vi "FGV Spans abarbeiten.vi"(5 "running":bool, 6 "Aktion":T10, 8 "error in (no error)":errorcluster caption="Fehler (Eingang, kein Fehler)", 11 "SpanInletClusterArray in":T1[](array[typedef]) {"zusätzliche Zeitdauer Erster Punkt" min=30 step=1 format="%#_5g"; "Zeitdauer Stufen" format="%#_5g"; "Max Fehler" format="%#_5g"; "Anzahl Stufen" format="%#_5g"; "Komponenten"."Komponente 5"."Komponente:" items=["NO (350,3000) LP 191C", "NO2 (150) LP 191C (1of2)", "NO2 (2000) LP 191C (2of2)", "N2O (300) LP 191C (1of2)", "NH3 (300) LP 191C (1of2)", "NH3 (900,3000) LP 191C (2of2)", "HNCO (400) 191C", "H2O% (30) LP 191C", "Formaldehyde (70,500) LP 191C", "CO2 low% (4) LP 191C (2of2)", "CO2% (20) LP 191C (1of2)", "CO (700) LP 191C (1of3)", "CO% (1) LP 191C (2of3)", "Propylene (1000) LP 191C", "Aromatic HC C7 (500) LP 191C", "Ethylene (1000) LP 191C", "CH4 (250) LP 191C (1of2)", "CH4 (5000) LP 191C (2of2)", "Ethane (1000) LP 191C", "Acetylene (1000) LP 191C", "HNO2 (20) 191C", "MeOH (1000) 191C", "CO% (10) LP 191C (3of3)", "Formic Acid (100) 191C", "SO2 (500) LP 191C", "Acetaldehyde (1000) LP 191C", "COS (100) LP 191C", "1,3 butadiene (100) LP 191C", "Oil as Octane (200) LP 191C", "N2O (1000) LP 191C (2of2)", "Propane (200) LP 191C", "NO2 autorange (2000)", "CO autorange (100000)", "CH4 autorange (5000)", "NH3 autorange (3000)", "Temp. Gascell", "Pressure Gascell", "sBeam@2500"]; "Komponenten"."Komponente 5"."Konzentration IST" format="%#.4f"; "Komponenten"."Komponente 5"."Genauigkeit" format="%#.1f"; "Komponenten"."Komponente 4"."Komponente:" items=["NO (350,3000) LP 191C", "NO2 (150) LP 191C (1of2)", "NO2 (2000) LP 191C (2of2)", "N2O (300) LP 191C (1of2)", "NH3 (300) LP 191C (1of2)", "NH3 (900,3000) LP 191C (2of2)", "HNCO (400) 191C", "H2O% (30) LP 191C", "Formaldehyde (70,500) LP 191C", "CO2 low% (4) LP 191C (2of2)", "CO2% (20) LP 191C (1of2)", "CO (700) LP 191C (1of3)", "CO% (1) LP 191C (2of3)", "Propylene (1000) LP 191C", "Aromatic HC C7 (500) LP 191C", "Ethylene (1000) LP 191C", "CH4 (250) LP 191C (1of2)", "CH4 (5000) LP 191C (2of2)", "Ethane (1000) LP 191C", "Acetylene (1000) LP 191C", "HNO2 (20) 191C", "MeOH (1000) 191C", "CO% (10) LP 191C (3of3)", "Formic Acid (100) 191C", "SO2 (500) LP 191C", "Acetaldehyde (1000) LP 191C", "COS (100) LP 191C", "1,3 butadiene (100) LP 191C", "Oil as Octane (200) LP 191C", "N2O (1000) LP 191C (2of2)", "Propane (200) LP 191C", "NO2 autorange (2000)", "CO autorange (100000)", "CH4 autorange (5000)", "NH3 autorange (3000)", "Temp. Gascell", "Pressure Gascell", "sBeam@2500"]; "Komponenten"."Komponente 4"."Konzentration IST" format="%#.4f"; "Komponenten"."Komponente 4"."Genauigkeit" format="%#.1f"; "Komponenten"."Komponente 3"."Komponente:" items=["NO (350,3000) LP 191C", "NO2 (150) LP 191C (1of2)", "NO2 (2000) LP 191C (2of2)", "N2O (300) LP 191C (1of2)", "NH3 (300) LP 191C (1of2)", "NH3 (900,3000) LP 191C (2of2)", "HNCO (400) 191C", "H2O% (30) LP 191C", "Formaldehyde (70,500) LP 191C", "CO2 low% (4) LP 191C (2of2)", "CO2% (20) LP 191C (1of2)", "CO (700) LP 191C (1of3)", "CO% (1) LP 191C (2of3)", "Propylene (1000) LP 191C", "Aromatic HC C7 (500) LP 191C", "Ethylene (1000) LP 191C", "CH4 (250) LP 191C (1of2)", "CH4 (5000) LP 191C (2of2)", "Ethane (1000) LP 191C", "Acetylene (1000) LP 191C", "HNO2 (20) 191C", "MeOH (1000) 191C", "CO% (10) LP 191C (3of3)", "Formic Acid (100) 191C", "SO2 (500) LP 191C", "Acetaldehyde (1000) LP 191C", "COS (100) LP 191C", "1,3 butadiene (100) LP 191C", "Oil as Octane (200) LP 191C", "N2O (1000) LP 191C (2of2)", "Propane (200) LP 191C", "NO2 autorange (2000)", "CO autorange (100000)", "CH4 autorange (5000)", "NH3 autorange (3000)", "Temp. Gascell", "Pressure Gascell", "sBeam@2500"]; "Komponenten"."Komponente 3"."Konzentration IST" format="%#.4f"; "Komponenten"."Komponente 3"."Genauigkeit" format="%#.1f"; "Komponenten"."Komponente 2"."Komponente:" items=["NO (350,3000) LP 191C", "NO2 (150) LP 191C (1of2)", "NO2 (2000) LP 191C (2of2)", "N2O (300) LP 191C (1of2)", "NH3 (300) LP 191C (1of2)", "NH3 (900,3000) LP 191C (2of2)", "HNCO (400) 191C", "H2O% (30) LP 191C", "Formaldehyde (70,500) LP 191C", "CO2 low% (4) LP 191C (2of2)", "CO2% (20) LP 191C (1of2)", "CO (700) LP 191C (1of3)", "CO% (1) LP 191C (2of3)", "Propylene (1000) LP 191C", "Aromatic HC C7 (500) LP 191C", "Ethylene (1000) LP 191C", "CH4 (250) LP 191C (1of2)", "CH4 (5000) LP 191C (2of2)", "Ethane (1000) LP 191C", "Acetylene (1000) LP 191C", "HNO2 (20) 191C", "MeOH (1000) 191C", "CO% (10) LP 191C (3of3)", "Formic Acid (100) 191C", "SO2 (500) LP 191C", "Acetaldehyde (1000) LP 191C", "COS (100) LP 191C", "1,3 butadiene (100) LP 191C", "Oil as Octane (200) LP 191C", "N2O (1000) LP 191C (2of2)", "Propane (200) LP 191C", "NO2 autorange (2000)", "CO autorange (100000)", "CH4 autorange (5000)", "NH3 autorange (3000)", "Temp. Gascell", "Pressure Gascell", "sBeam@2500"]; "Komponenten"."Komponente 2"."Konzentration IST" format="%#.4f"; "Komponenten"."Komponente 2"."Genauigkeit" format="%#.1f"; "Komponenten"."Komponente 1"."Komponente:" items=["NO (350,3000) LP 191C", "NO2 (150) LP 191C (1of2)", "NO2 (2000) LP 191C (2of2)", "N2O (300) LP 191C (1of2)", "NH3 (300) LP 191C (1of2)", "NH3 (900,3000) LP 191C (2of2)", "HNCO (400) 191C", "H2O% (30) LP 191C", "Formaldehyde (70,500) LP 191C", "CO2 low% (4) LP 191C (2of2)", "CO2% (20) LP 191C (1of2)", "CO (700) LP 191C (1of3)", "CO% (1) LP 191C (2of3)", "Propylene (1000) LP 191C", "Aromatic HC C7 (500) LP 191C", "Ethylene (1000) LP 191C", "CH4 (250) LP 191C (1of2)", "CH4 (5000) LP 191C (2of2)", "Ethane (1000) LP 191C", "Acetylene (1000) LP 191C", "HNO2 (20) 191C", "MeOH (1000) 191C", "CO% (10) LP 191C (3of3)", "Formic Acid (100) 191C", "SO2 (500) LP 191C", "Acetaldehyde (1000) LP 191C", "COS (100) LP 191C", "1,3 butadiene (100) LP 191C", "Oil as Octane (200) LP 191C", "N2O (1000) LP 191C (2of2)", "Propane (200) LP 191C", "NO2 autorange (2000)", "CO autorange (100000)", "CH4 autorange (5000)", "NH3 autorange (3000)", "Temp. Gascell", "Pressure Gascell", "sBeam@2500"]; "Komponenten"."Komponente 1"."Konzentration IST" format="%#.4f"; "Komponenten"."Komponente 1"."Genauigkeit" format="%#.1f"; "Ablaufdatum" format="%<%d.%m.%Y>T"; "Gasflasche" items=["----"=10000, "IAG NH3 3000"=0, "IAG NH3 200"=1, "IAG NH3 2000"=2, "IAG MG"=3, "IAG O2"=4]}) -> (0 "error out":errorcluster caption="Fehler (Ausgang)", 1 "Comp Idx out":i32, 2 "start":bool, 3 "active SPAN Idx out":i32, 4 "running out":bool, 7 "Zeitstempel":timestamp)   [LabVIEW 2020, in "Linearisierung v2.lvlib" / "SpanEinstellungen.lvlib"]
uses:
  SpanEinstellungen.lvlib
  Aktion FGV Spans abarbeiten.ctl
  SpanInletCluster.ctl
  Seiten/System Einstellungen V2/Konfig Gasflasche.ctl
  Seiten/System Einstellungen V2/Analysatoren.ctl
  Seiten/System Einstellungen V2/Gasflasche Auswahl.ctl
  Komponentencluster mit Formel.ctl
  Komponentenauswahl mit Formel.ctl
  Visualisierungs Elemente/String - Eingabefeld.ctl
  Einheit.ctl
  Seiten/System Einstellungen V2/Traegergas.ctl
  Seiten/System Einstellungen V2/System Einstellungen V2.lvlib
panel:
  # "sec"
  # "%"
  # "sec"
  # "Komponente"
  # "Formel"
  # "Konzentration"
  # "Einheit"
  # "Genauigkeit [%]"
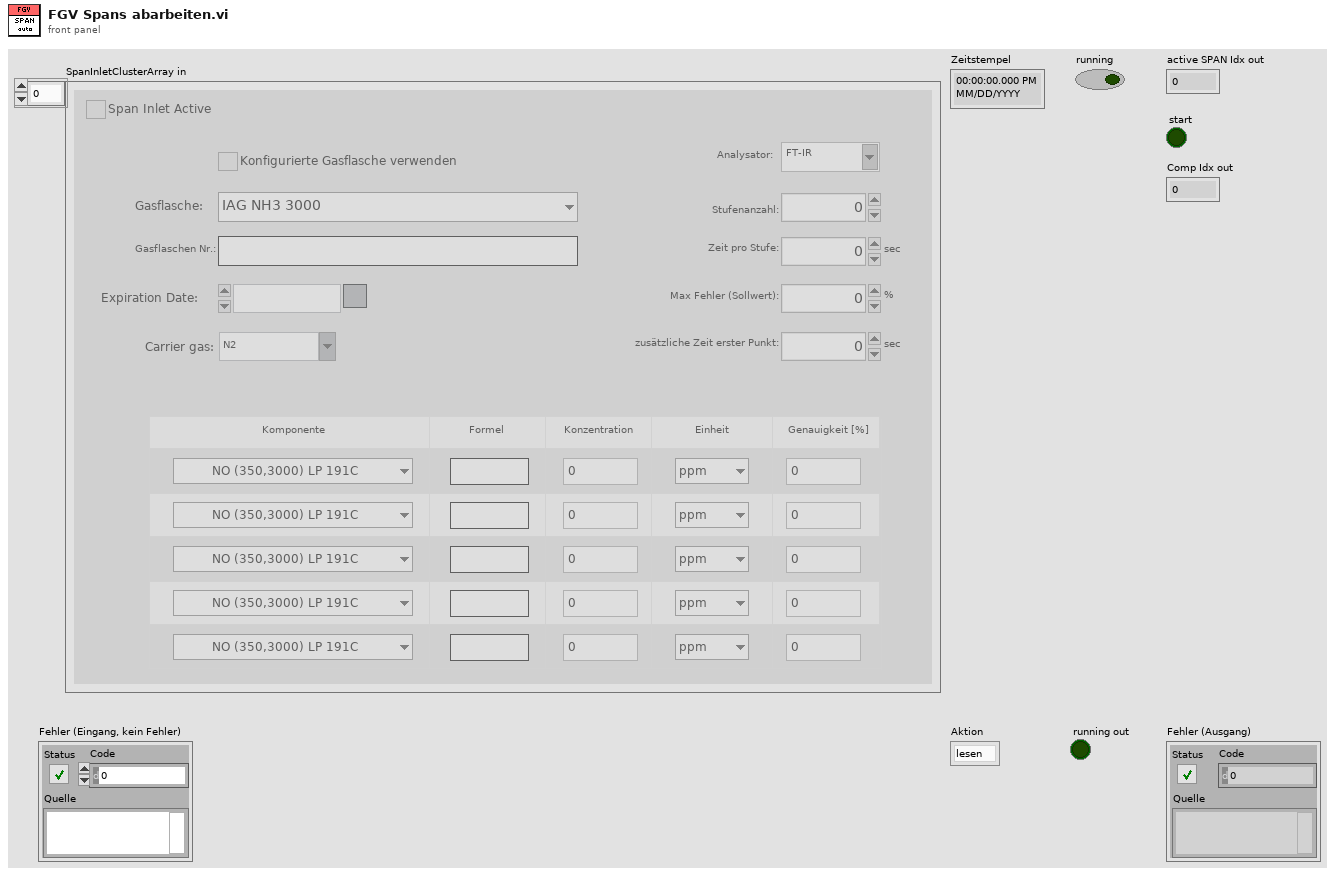
[diagram p1: front panel]
types:
  T1 = typedef "Linearisierung v2.lvlib/SpanEinstellungen.lvlib/SpanInletCluster.ctl" = cluster{"Span Inlet Active":T2, "Analysator":T3, "Konfig Gasflasche":T2, "Gasflasche":T4, "Gasflaschen Nr.:":string, "Ablaufdatum":timestamp, "Komponenten":T5, "Zeitdauer Stufen":sgl, "Max Fehler":sgl, "Anzahl Stufen":sgl, "Trägergas":T9, "zusätzliche Zeitdauer Erster Punkt":sgl}
  T2 = typedef "System Einstellungen V2.lvlib/Konfig Gasflasche.ctl" = bool
  T3 = typedef "System Einstellungen V2.lvlib/Analysatoren.ctl" = string
  T4 = typedef "System Einstellungen V2.lvlib/Gasflasche Auswahl.ctl" = u16
  T5 = typedef "Linearisierung v2.lvlib/SpanEinstellungen.lvlib/Komponentencluster mit Formel.ctl" = cluster{"Komponente 1":T6, "Komponente 2":T6, "Komponente 3":T6, "Komponente 4":T6, "Komponente 5":T6}
  T6 = typedef "Linearisierung v2.lvlib/SpanEinstellungen.lvlib/Komponentenauswahl mit Formel.ctl" = cluster{"Komponente:":u16, "Summenformel":T7, "Konzentration IST":dbl, "Einheit":T8, "Genauigkeit":dbl}
  T7 = typedef "String - Eingabefeld.ctl" = string
  T8 = typedef "Linearisierung v2.lvlib/SpanEinstellungen.lvlib/Einheit.ctl" = enum16{"ppm", "%"}
  T9 = typedef "System Einstellungen V2.lvlib/Traegergas.ctl" = string
  T10 = typedef "Linearisierung v2.lvlib/SpanEinstellungen.lvlib/Aktion FGV Spans abarbeiten.ctl" = enum16{"lesen", "idle", "start", "next", "comp", "init", "running", "abort"}
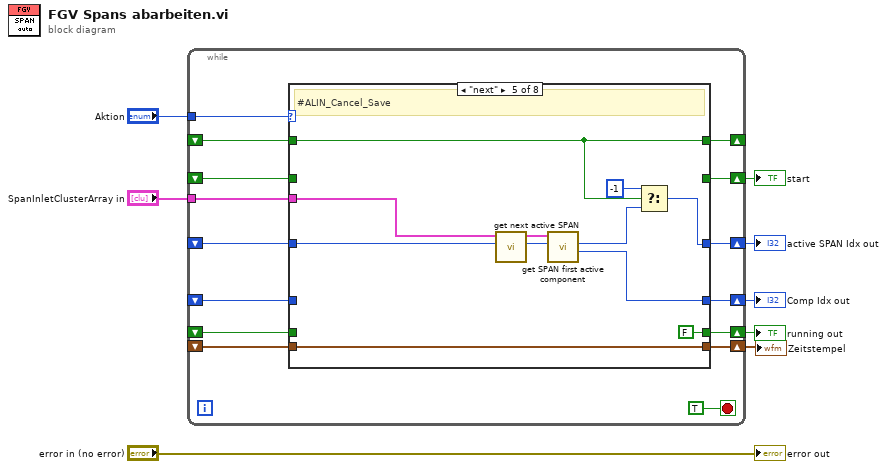
[diagram p0: block diagram]
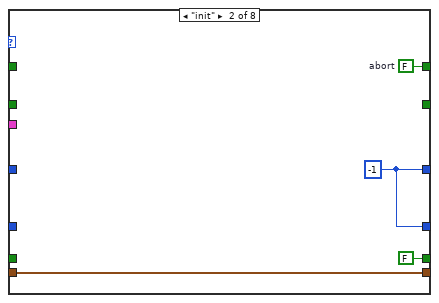
[diagram p3: hidden frame]
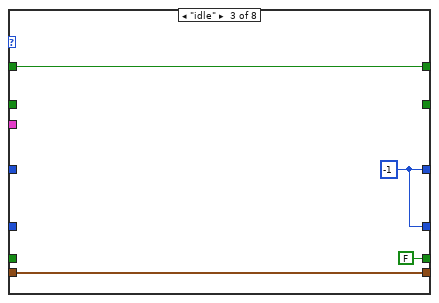
[diagram p4: hidden frame]
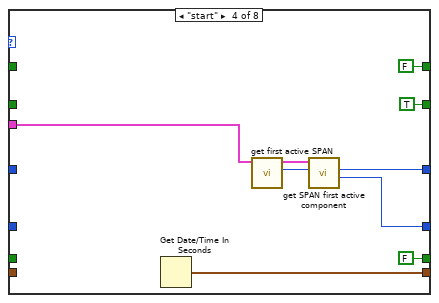
[diagram p5: hidden frame]
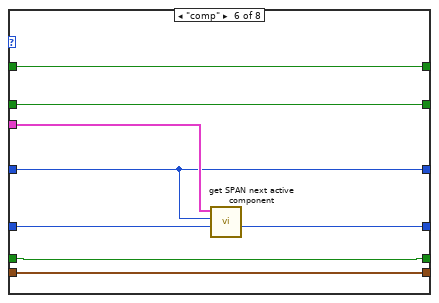
[diagram p6: hidden frame]
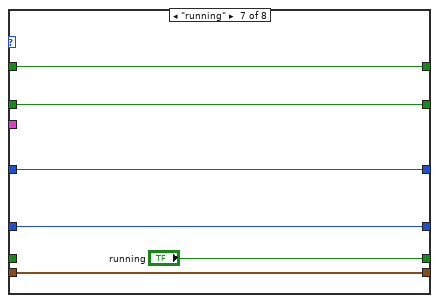
[diagram p7: hidden frame]
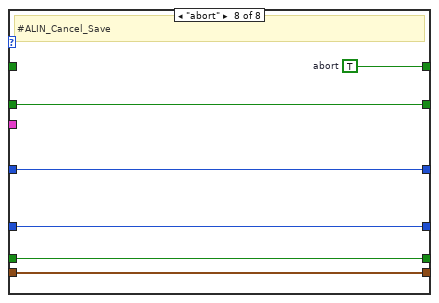
[diagram p8: hidden frame]
diagram:
  n1 = while {
    tunnel: "Aktion" -> [w22]
    shift-right: [w20] -> w7
    shift-left: _ -> [w21]
    shift-right: [w18] -> w6
    shift-left: _ -> [w19]
    tunnel: "SpanInletClusterArray in" -> [w17]
    shift-right: [w16] -> w3
    shift-left: _ -> [w15]
    shift-right: [w14] -> w2
    shift-left: _ -> [w13]
    shift-right: [w12] -> w1
    shift-left: _ -> [w11]
    shift-right: [w10] -> _
    shift-left: _ -> [w9]
    stop <- TRUE stop-if-true
    n2 = case shown="\"next\"" w22 {
      tunnel: w21 -> [w29 _ _ _ w55 w61 w71 w77]
      tunnel: [w29 w33 w37 w40 w47 w61 w71 w77] -> w20
      tunnel: w19 -> [w28 _ _ _ _ w64 w70 w76]
      tunnel: [w28 w33 w37 w42 w51 w60 w70 w76] -> w18
      tunnel: w17 -> [_ _ _ w46 w57 w65 _ _]
      tunnel: [w27 FALSE ("running") FALSE ("running") FALSE ("running") FALSE ("running") w63 "running" w75] -> w16
      tunnel: w15 -> [w27 _ _ _ _ w63 _ w75]
      tunnel: [w26 w31 w35 w44 w54 w62 w68 w74] -> w14
      tunnel: w13 -> [w26 w31 w35 _ w54 w62 w68 w74]
      tunnel: [w25 _ _ TRUE ("running") _ w59 w67 w73] -> w12
      tunnel: w11 -> [w25 _ _ _ _ w59 w67 w73]
      tunnel: [w24 w30 w34 FALSE ("abort") w50 w58 w66 w72] -> w10
      tunnel: w9 -> [w24 _ w34 _ w50 w58 w66 _]
      frame "lesen", Default {
      }
      frame "init" {
        w30 = FALSE  # abort
        w33 = -1 ("Index next active SPAN")
      }
      frame "idle" {
        w37 = -1 ("SPAN Idx")
      }
      frame "start" {
        n3 = Get Date/Time In Seconds() -> (seconds since 1Jan1904=w44:timestamp)
        n4 = call "get first active SPAN.vi"("SpanInletClusterArray in"=w46) -> ("Index first active SPAN"=w43:i32, "SpanInletClusterArray out"=w41:T1[])  [unwired: 8 in, 1 out]
        n5 = call "get SPAN first active component.vi"("SPAN Idx"=w43, "SpanInletClusterArray in"=w41) -> ("first aktive Komponente"=w42:i32, "SPAN Idx out"=w40:i32)  [unwired: 6 in, 2 out]
      }
      frame "next" {
        # "#ALIN_Cancel_Save"
        n6 = call "get next active SPAN.vi"("Index active SPAN"=w55, "SpanInletClusterArray in"=w57) -> ("Index next active SPAN"=w52:i32, "SpanInletClusterArray out"=w53:T1[])  [unwired: 7 in, 1 out]
        n7 = call "get SPAN first active component.vi"("SPAN Idx"=w52, "SpanInletClusterArray in"=w53) -> ("first aktive Komponente"=w51:i32, "SPAN Idx out"=w49:i32)  [unwired: 6 in, 2 out]
        n8 = Select(t=-1 ("f"), s=w50, f=w49) -> (s? t:f=w47:i32)
      }
      frame "comp" {
        n9 = call "get SPAN next active component.vi"("Komponente Idx"=w64, "SPAN Idx"=w61, "SpanInletClusterArray in"=w65) -> ("next aktive Komponente"=w60:i32)  [unwired: 6 in, 2 out]
      }
      frame "running" {
      }
      frame "abort" {
        w72 = TRUE  # abort
        # "#ALIN_Cancel_Save"
      }
    }
  }
  "active SPAN Idx out" <- w7
  "Comp Idx out" <- w6
  "running out" <- w3
  "Zeitstempel" <- w2
  "start" <- w1
  "error out" <- "error in (no error)"
